vi "测试1.vi"() -> ()   [LabVIEW 2016]
panel:
  in  "选择菜单":u16(ring) items=["醇黑浓情系列奶茶", "醇香奶茶"]
  in  "规格":u16(ring) items=["大杯", "小杯", "中杯"]
  in  "选择奶茶":u16(ring) items=["巧克力可可", "燕麦巧克力"]
  out "价格":dbl
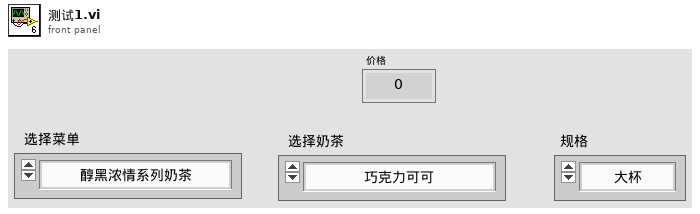
[diagram p1: front panel]
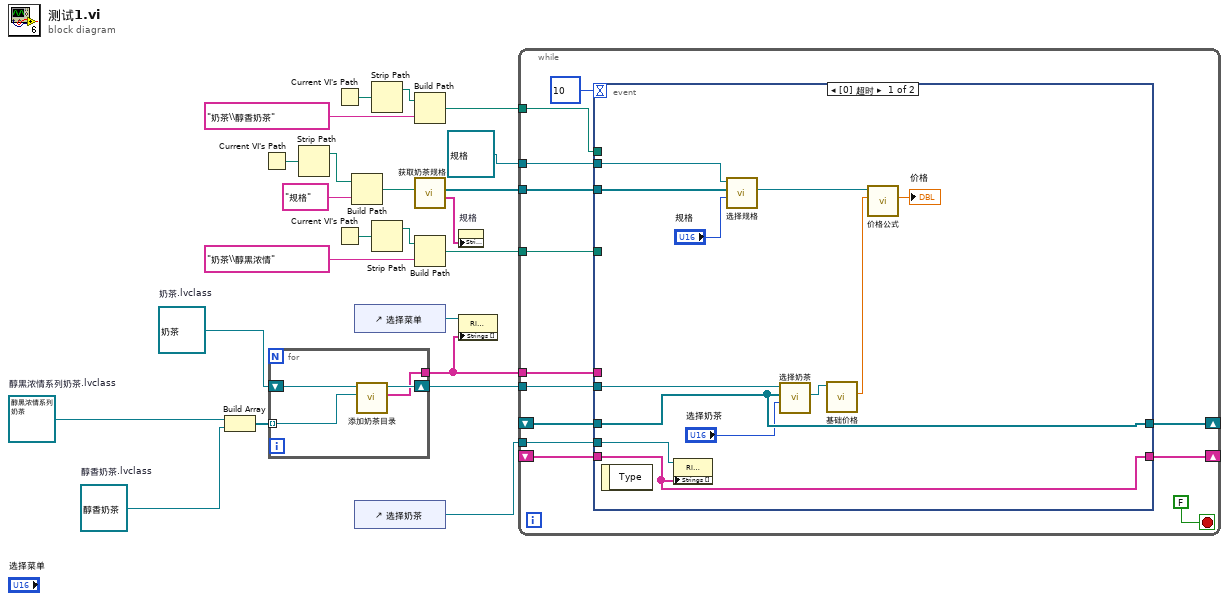
[diagram p0: block diagram]
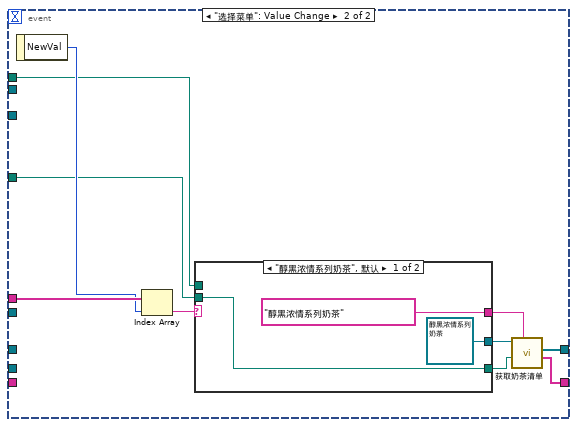
[diagram p2: hidden frame]
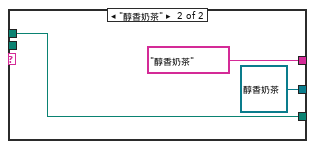
[diagram p3: hidden frame]
diagram:
  w21 = refnum<class "醇香奶茶.lvclass"> refnum  # 醇香奶茶.lvclass
  w22 = refnum<class "醇黑浓情系列奶茶.lvclass"> refnum  # 醇黑浓情系列奶茶.lvclass
  w23 = refnum<class "奶茶.lvclass"> refnum  # 奶茶.lvclass
  n1 = Build Array(w22, w21) -> (w20:refnum<class "奶茶.lvclass">[])
  n2 = Current VI's Path() -> (path=w6:path)
  n3 = for {
    tunnel: w20 -> [w26] mode=indexing
    shift-right: [w25] -> w15
    shift-left: w23 -> [w27]
    tunnel: [w24] -> w18
    n4 = call "添加奶茶目录.vi"("奶茶.lvclass"=w26, "奶茶 输入"=w27) -> ("奶茶目录名称"=w24:string[], "奶茶 输出"=w25:refnum<class "奶茶.lvclass">)  [unwired: 7 in, 1 out]
  }
  n5 = Strip Path(path=w6) -> (stripped path=w5:path)  [unwired: 1 out]
  n6 = Current VI's Path() -> (path=w2:path)
  n7 = Current VI's Path() -> (path=w12:path)
  n8 = Build Path(base path=w5, name or relative path="规格" ("名称或相对路径")) -> (appended path=w3:path)
  n9 = control-ref of="选择菜单"() -> (w19:refnum<vi>)
  n10 = control-ref of="选择奶茶"() -> (w17:refnum<vi>)
  n11 = Strip Path(path=w2) -> (stripped path=w1:path)  [unwired: 1 out]
  n12 = Strip Path(path=w12) -> (stripped path=w9:path)  [unwired: 1 out]
  n13 = Build Path(base path=w1, name or relative path="奶茶\\醇香奶茶" ("名称或相对路径")) -> (appended path=w10:path)
  n14 = call "获取奶茶规格.vi"("Folder Path"=w3) -> ("清单名称"=w13:string[], "规格"=w14:refnum<class>[])  [unwired: 9 in]
  n15 = Build Path(base path=w9, name or relative path="奶茶\\醇黑浓情" ("名称或相对路径")) -> (appended path=w7:path)
  n16 = property on="规格" class="Ring (严格)"("Strings []"=w13) -> ()  [unwired: 2 in, 2 out]
  n17 = property on="属性节点" class="Ring (严格)"(reference=w19, "Strings []"=w18) -> ()  [unwired: 1 in, 2 out]
  n18 = while {
    tunnel: w10 -> [w39]
    tunnel: w18 -> [w38]
    shift-right: [w37] -> _
    shift-left: _ -> [w34]
    shift-right: [w36] -> _
    shift-left: _ -> [w35]
    tunnel: w17 -> [w33]
    tunnel: w7 -> [w32]
    tunnel: w14 -> [w30]
    tunnel: refnum<class "规格.lvclass"> refnum ("规格.lvclass") -> [w29]
    tunnel: w15 -> [w28]
    stop <- FALSE stop-if-true
    n19 = event shown="[0] 超时" {
      selector: _ -> [_ _]
      dyn-events: _ -> [_ _]
      timeout: 10 -> [_ _]
      tunnel: w39 -> [_ w54]
      tunnel: w38 -> [_ w62]
      tunnel: [w51 w58] -> w37
      tunnel: [w46 w57] -> w36
      tunnel: w35 -> [w46 _]
      tunnel: w34 -> [w51 _]
      tunnel: w33 -> [w52 _]
      tunnel: w32 -> [_ w53]
      tunnel: w30 -> [w49 _]
      tunnel: w29 -> [w50 _]
      tunnel: w28 -> [w43 _]
      event Timeout {
        n20 = event-data() -> ()  [unwired: 1 in, 1 out]
        n21 = property on="属性节点" class="Ring (严格)"(reference=w52, "Strings []"=w51) -> ()  [unwired: 1 in, 2 out]
        n22 = call "选择规格.vi"("索引"="规格", "规格"=w49, "规格 输入"=w50) -> ("特定类引用"=w48:refnum<class "规格.lvclass">)  [unwired: 6 in, 2 out]
        n23 = call "选择奶茶.vi"("数值"="选择奶茶", "奶茶清单"=w46, "奶茶 输入"=w43) -> ("选择的奶茶"=w45:refnum<class "奶茶.lvclass">)  [unwired: 6 in, 2 out]
        n24 = call-dynamic "基础价格.vi"("奶茶 输入"=w45) -> ("基础价格"=w44:dbl)  [unwired: 8 in, 2 out]
        n25 = call-dynamic "价格公式.vi"("基础价格"=w44, "规格 输入"=w48) -> ("价格"=→"价格":dbl)  [unwired: 7 in, 2 out]
      }
      event "选择菜单": Value Change {
        n26 = event-data() -> ("NewVal"=w61:u16)  [unwired: 1 in]
        n27 = Index Array(array=w62, index=w61) -> (element=w60:string)
        n28 = case shown="\"醇黑浓情系列奶茶\", 默认" w60 {
          tunnel: [refnum<class "醇黑浓情系列奶茶.lvclass"> refnum ("醇黑浓情系列奶茶.lvclass") refnum<class "醇香奶茶.lvclass"> refnum ("醇香奶茶.lvclass")] -> w59
          tunnel: ["醇黑浓情系列奶茶" ("父类") "醇香奶茶" ("父类")] -> w56
          tunnel: [w63 w66] -> w55
          tunnel: w54 -> [_ w66]
          tunnel: w53 -> [w63 _]
          frame "醇黑浓情系列奶茶", Default {
          }
          frame "醇香奶茶" {
          }
        }
        n29 = call-dynamic "获取奶茶清单.vi"("父类"=w56, "Folder Path"=w55, "奶茶 输入"=w59) -> ("清单名称"=w58:string[], "数组"=w57:refnum<class>[])  [unwired: 5 in, 2 out]
      }
    }
  }
